vi "4FileHeaderWrite.vi"(8 "MetaData Cluster":T1, 10 "In Use Cluster":T2) -> (2 "Cluster out":T3)   [LabVIEW 2014]
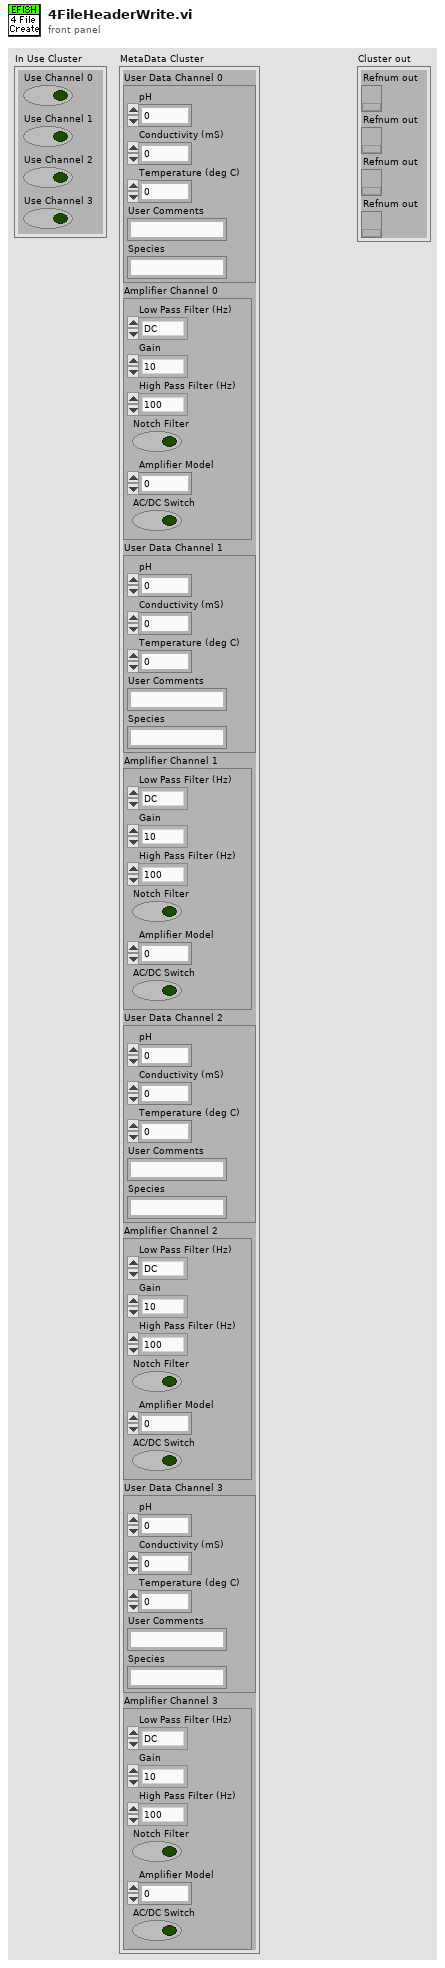
[diagram p1: front panel]
types:
  T1 = cluster{"User Data Channel 0":cluster{"pH":dbl, "Conductivity (mS)":dbl, "Temperature (deg C)":dbl, "User Comments":string, "Species":string}, "Amplifier Channel 0":cluster{"Low Pass Filter (Hz)":enum16{"DC", "0.1", "1", "3", "10", "30", "100", "300"}, "Gain ":enum16{"10", "20", "50", "100", "200", "500", "1000", "2k", "5k", "10k", "20k", "50k"}, "High Pass Filter (Hz)":enum16{"100", "500", "1000", "3000", "5000", "10,000", "20,000", "30,000", "50,000"}, "Notch Filter":bool, "Amplifier Model":u16, "AC/DC Switch":bool}, "User Data Channel 1":cluster{"pH":dbl, "Conductivity (mS)":dbl, "Temperature (deg C)":dbl, "User Comments":string, "Species":string}, "Amplifier Channel 1":cluster{"Low Pass Filter (Hz)":enum16{"DC", "0.1", "1", "3", "10", "30", "100", "300"}, "Gain ":enum16{"10", "20", "50", "100", "200", "500", "1000", "2k", "5k", "10k", "20k", "50k"}, "High Pass Filter (Hz)":enum16{"100", "500", "1000", "3000", "5000", "10,000", "20,000", "30,000", "50,000"}, "Notch Filter":bool, "Amplifier Model":u16, "AC/DC Switch":bool}, "User Data Channel 2":cluster{"pH":dbl, "Conductivity (mS)":dbl, "Temperature (deg C)":dbl, "User Comments":string, "Species":string}, "Amplifier Channel 2":cluster{"Low Pass Filter (Hz)":enum16{"DC", "0.1", "1", "3", "10", "30", "100", "300"}, "Gain ":enum16{"10", "20", "50", "100", "200", "500", "1000", "2k", "5k", "10k", "20k", "50k"}, "High Pass Filter (Hz)":enum16{"100", "500", "1000", "3000", "5000", "10,000", "20,000", "30,000", "50,000"}, "Notch Filter":bool, "Amplifier Model":u16, "AC/DC Switch":bool}, "User Data Channel 3":cluster{"pH":dbl, "Conductivity (mS)":dbl, "Temperature (deg C)":dbl, "User Comments":string, "Species":string}, "Amplifier Channel 3":cluster{"Low Pass Filter (Hz)":enum16{"DC", "0.1", "1", "3", "10", "30", "100", "300"}, "Gain ":enum16{"10", "20", "50", "100", "200", "500", "1000", "2k", "5k", "10k", "20k", "50k"}, "High Pass Filter (Hz)":enum16{"100", "500", "1000", "3000", "5000", "10,000", "20,000", "30,000", "50,000"}, "Notch Filter":bool, "Amplifier Model":u16, "AC/DC Switch":bool}}
  T2 = cluster{"Use Channel 0":bool, "Use Channel 1":bool, "Use Channel 2":bool, "Use Channel 3":bool}
  T3 = cluster{"Refnum out":refnum<k34>, "Refnum out":refnum<k34>, "Refnum out":refnum<k34>, "Refnum out":refnum<k34>}
  T4 = cluster{"pH":dbl, "Conductivity (mS)":dbl, "Temperature (deg C)":dbl, "User Comments":string, "Species":string}
  T5 = cluster{"Low Pass Filter (Hz)":enum16{"DC", "0.1", "1", "3", "10", "30", "100", "300"}, "Gain ":enum16{"10", "20", "50", "100", "200", "500", "1000", "2k", "5k", "10k", "20k", "50k"}, "High Pass Filter (Hz)":enum16{"100", "500", "1000", "3000", "5000", "10,000", "20,000", "30,000", "50,000"}, "Notch Filter":bool, "Amplifier Model":u16, "AC/DC Switch":bool}
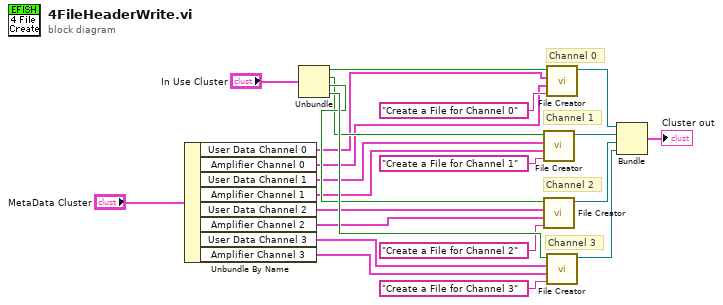
[diagram p0: block diagram]
diagram:
  # "Channel 3"
  # "Channel 2"
  # "Channel 1"
  # "Channel 0"
  n1 = Unbundle By Name("MetaData Cluster") -> ("User Data Channel 0"=w10:T4, "Amplifier Channel 0"=w9:T5, "User Data Channel 1"=w8:T4, "Amplifier Channel 1"=w7:T5, "User Data Channel 2"=w6:T4, "Amplifier Channel 2"=w5:T5, "User Data Channel 3"=w4:T4, "Amplifier Channel 3"=w3:T5)
  n2 = Unbundle("In Use Cluster") -> ("Use Channel 0"=w13:bool, "Use Channel 1"=w14:bool, "Use Channel 2"=w15:bool, "Use Channel 3"=w16:bool)
  n3 = call "File Creator.vi"("prompt"="Create a File for Channel 1", "Amplifier Channel 1"=w7, "User Data Channel 1"=w8, "Use Channel in"=w14) -> ("Refnum out"=w18:refnum<k34>)  [unwired: 7 in]
  n4 = call "File Creator.vi"("prompt"="Create a File for Channel 2", "Amplifier Channel 1"=w5, "User Data Channel 1"=w6, "Use Channel in"=w15) -> ("Refnum out"=w19:refnum<k34>)  [unwired: 7 in]
  n5 = call "File Creator.vi"("prompt"="Create a File for Channel 0", "Amplifier Channel 1"=w9, "User Data Channel 1"=w10, "Use Channel in"=w13) -> ("Refnum out"=w17:refnum<k34>)  [unwired: 7 in]
  n6 = call "File Creator.vi"("prompt"="Create a File for Channel 3", "Amplifier Channel 1"=w3, "User Data Channel 1"=w4, "Use Channel in"=w16) -> ("Refnum out"=w20:refnum<k34>)  [unwired: 7 in]
  n7 = Bundle("Refnum out"=w17, "Refnum out"=w18, "Refnum out"=w19, "Refnum out"=w20) -> (→"Cluster out":T3)  [unwired: 1 in]
